vi "Visualize_Results_of_Filtering_wt_Cross-1.vi"(7 "[IN] Number of event":i8=2, 8 "error IN":errorcluster, 9 "[IN] Localization Settings":T5 {"[IN] Image Type" items=["Grayscale (U8)", "Grayscale (I16)", "Grayscale (SGL)", "Complex (CSG)", "RGB (U32)", "HSL (U32)", "RGB (U64)", "Grayscale (U16)"]; "[IN] Particle Filter Setups"."Type of particle filter"."Measurement Parameter" items=["Center of Mass X", "Center of Mass Y", "First Pixel X", "First Pixel Y", "Bounding Rect Left", "Bounding Rect Top", "Bounding Rect Right", "Bounding Rect Bottom", "Max Feret Diameter Start X", "Max Feret Diameter Start Y", "Max Feret Diameter End X", "Max Feret Diameter End Y", "Max Horiz. Segment Length Left", "Max Horiz. Segment Length Right", "Max Horiz. Segment Length Row", "-", "Bounding Rect Width", "Bounding Rect Height", "Bounding Rect Diagonal", "Perimeter", "Convex Hull Perimeter", "Holes' Perimeter", "Max Feret Diameter", "Equivalent Ellipse Major Axis", "Equivalent Ellipse Minor Axis", "Equivalent Ellipse Minor Axis (Feret)", "Equivalent Rect Long Side", "Equivalent Rect Short Side", "Equivalent Rect Diagonal", "Equivalent Rect Short Side (Feret)", "Average Horiz. Segment Length", "Average Vert. Segment Length", "Hydraulic Radius", "Waddel Disk Diameter", "-", "Area", "Holes' Area", "Particle & Holes' Area", "Convex Hull Area", "Image Area", "-", "Number of Holes", "Number of Horiz. Segments", "Number of Vert. Segments", "-", "Orientation", "Max Feret Diameter Orientation", "-", "% Area/Image Area", "% Area/(Particle & Holes' Area)", "Ratio of Equivalent Ellipse Axes", "Ratio of Equivalent Rect Sides", "-", "Elongation Factor", "Compactness Factor", "Heywood Circularity Factor", "Type Factor", "-", "Sum X", "Sum Y", "Sum XX", "Sum XY", "Sum YY", "Sum XXX", "Sum XXY", "Sum XYY", "Sum YYY", "-", "Moment of Inertia XX", "Moment of Inertia XY", "Moment of Inertia YY", "Moment of Inertia XXX", "Moment of Inertia XXY", "Moment of Inertia XYY", "Moment of Inertia YYY", "Norm. Moment of Inertia XX", "Norm. Moment of Inertia XY", "Norm. Moment of Inertia YY", "Norm. Moment of Inertia XXX", "Norm. Moment of Inertia XXY", "Norm. Moment of Inertia XYY", "Norm. Moment of Inertia YYY", "Hu Moment 1", "Hu Moment 2", "Hu Moment 3", "Hu Moment 4", "Hu Moment 5", "Hu Moment 6", "Hu Moment 7"]}, 10 "# Frame":u32 max=499, 11 "[IN] Images Array":T1[](array[typedef])) -> (0 "error OUT":errorcluster, 2 "[OUT] LoG with Particles":T1)   [LabVIEW 2013]
uses:
  <vilib>/vision/Image Controls.llb/IMAQ Image.ctl
  <vilib>/vision/Avi.llb/IMAQ AVI2 Refnum.ctl
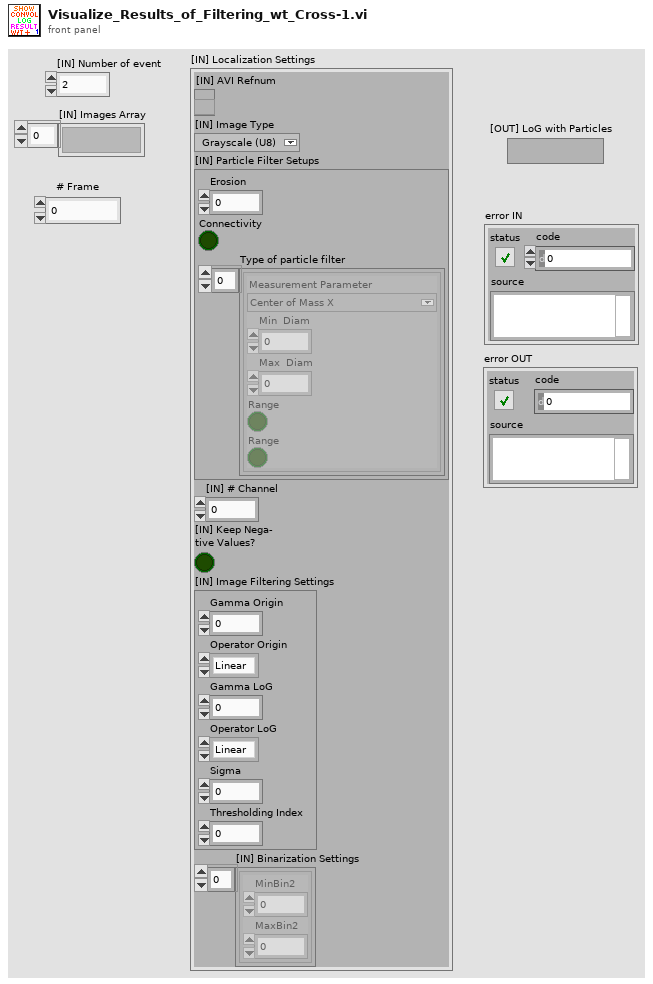
[diagram p1: front panel]
types:
  T1 = typedef "IMAQ Image.ctl" = refnum<image>
  T2 = typedef "IMAQ AVI2 Refnum.ctl" = refnum<k20>
  T3 = typedef "Image Type" = u32
  T4 = typedef "Particle Parameters" = i32
  T5 = cluster{"[IN] AVI Refnum":T2, "[IN] Image Type":T3, "[IN] Particle Filter Setups":cluster{"Erosion":i32, "Connectivity ":bool, "Type of particle filter":cluster{"Measurement Parameter":T4, "Min  Diam":dbl, "Max  Diam":dbl, "Range":bool, "Range":bool}[]}, "[IN] # Channel":u8, "[IN] Keep Nega-\ntive Values?":bool, "[IN] Image Filtering Settings":cluster{"Gamma Origin":sgl, "Operator Origin":enum32{"Linear", "Log", "Exp", "Square", "Square root", "Power X", "Power 1/X"}, "Gamma LoG":sgl, "Operator LoG":enum32{"Linear", "Log", "Exp", "Square", "Square root", "Power X", "Power 1/X"}, "Sigma":dbl, "Thresholding Index":i8}, "[IN] Binarization Settings":cluster{"MinBin2":sgl, "MaxBin2":sgl}[]}
  T6 = cluster{"Gamma Origin":sgl, "Operator Origin":enum32{"Linear", "Log", "Exp", "Square", "Square root", "Power X", "Power 1/X"}, "Gamma LoG":sgl, "Operator LoG":enum32{"Linear", "Log", "Exp", "Square", "Square root", "Power X", "Power 1/X"}, "Sigma":dbl, "Thresholding Index":i8}
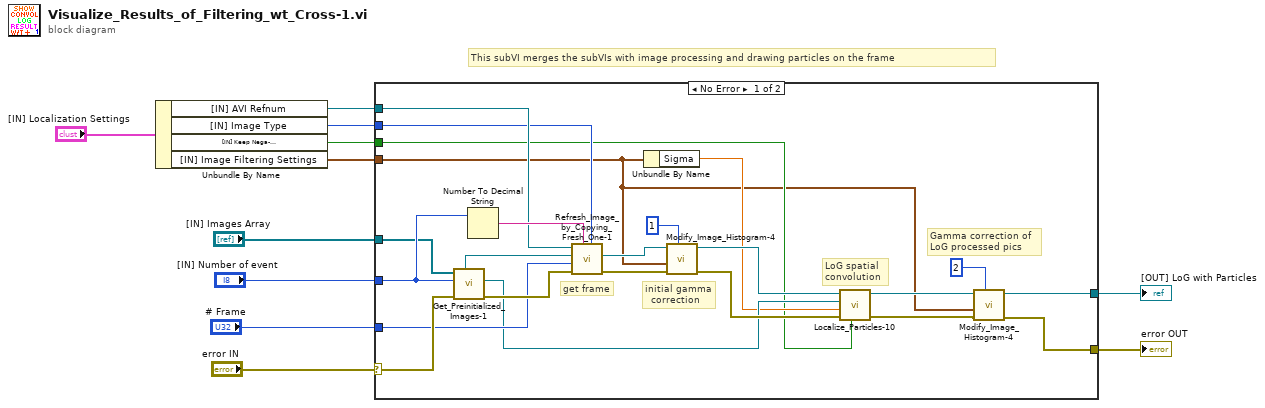
[diagram p0: block diagram]
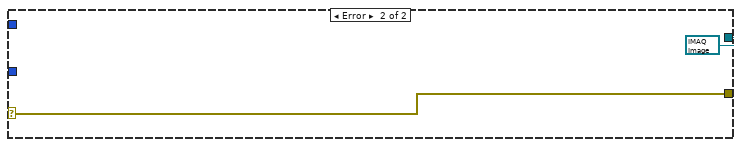
[diagram p2: hidden frame]
diagram:
  # "This subVI merges the subVIs with image processing and drawing particles on the frame"
  n1 = Unbundle By Name("[IN] Localization Settings") -> ("[IN] AVI Refnum"=w2:T2, "[IN] Image Type"=w1:T3, "[IN] Keep Nega-\ntive Values?"=w5:bool, "[IN] Image Filtering Settings"=w4:T6)
  n2 = case shown="No Error" "error IN" {
    selector: "error IN" -> [w31 w36]
    tunnel: [w12 w36] -> w10
    tunnel: "[IN] Number of event" -> [w30 _]
    tunnel: "# Frame" -> [w28 _]
    tunnel: "[IN] Images Array" -> [w29 _]
    tunnel: w2 -> [w27 _]
    tunnel: w1 -> [w26 _]
    tunnel: w5 -> [w18 _]
    tunnel: w4 -> [w15 _]
    tunnel: [w13 T1 refnum ("[OUT] Binarized Image")] -> w3
    frame No Error {
      # "Gamma correction of \nLoG processed pics"
      # "LoG spatial\nconvolution"
      # "initial gamma\n  correction"
      # "get frame"
      n3 = call "Get_Preinitialized_Images-1.vi"("error IN"=w31, "[IN] Number of event"=w30, "[IN] Images Array"=w29) -> ("error OUT"=w34:errorcluster, "[OUT] Processed Image #1"=w20:T1, "[OUT] Source Image #1"=w33:T1)  [unwired: 1 in, 2 out]
      n4 = Number To Decimal String(number=w30) -> (decimal integer string=w32:string)  [unwired: 1 in]
      n5 = call "Refresh_Image_by_Copying_Fresh_One-1.vi"("[IN] Image Type"=w26, "[IN] Unique ID\n(# of Event)"=w32, "error IN"=w34, "Frame Number"=w28, "[IN] Preinitialized Image"=w33, "[IN] AVI Refnum"=w27) -> ("error OUT"=w23:errorcluster, "[OUT] Frame"=w21:T1)  [unwired: 1 in, 1 out]
      n6 = Unbundle By Name(w15) -> ("Sigma"=w19:dbl)
      n7 = call "Modify_Image_Histogram-4.vi"("1 - Origin\n2 - LoG"=u8 1 ("# channel"), "error IN"=w23, "[IN] Image Filtering Settings"=w15, "[IN] LoG Processed Image"=w21) -> ("error OUT"=w24:errorcluster, "[OUT] Histogram Modified Image"=w25:T1)  [unwired: 5 in, 1 out]
      n8 = call "Localize_Particles-10.vi"("Keep Nega-\ntive Values?"=w18, "error IN"=w24, "[IN] Sigma"=w19, "[IN] Destination Image"=w20, "[IN] Frame"=w25) -> ("error OUT"=w16:errorcluster, "[OUT] LoG Processed Image"=w17:T1)  [unwired: 3 in, 1 out]
      n9 = call "Modify_Image_Histogram-4.vi"("1 - Origin\n2 - LoG"=u8 2 ("# channel"), "error IN"=w16, "[IN] Image Filtering Settings"=w15, "[IN] LoG Processed Image"=w17) -> ("error OUT"=w12:errorcluster, "[OUT] Histogram Modified Image"=w13:T1)  [unwired: 5 in, 1 out]
    }
    frame Error {
    }
  }
  "error OUT" <- w10
  "[OUT] LoG with Particles" <- w3
